vi "Test init device.vi"() -> ()   [LabVIEW 2020]
uses:
  PIC-device/PIC-Device.lvclass
  Toggle 6/Toggle 6.lvclass
  C:/Sandbox/RF Bench/Source Code/WiSpry Test Framework/Devices/PIC-device/PIC-Device.lvclass
panel:
  out "Device out":refnum<class "PIC-Device.lvclass">
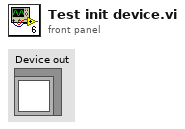
[diagram p1: front panel]
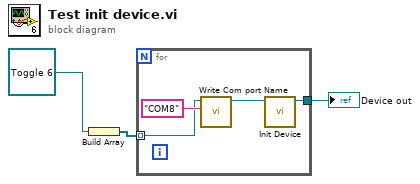
[diagram p0: block diagram]
diagram:
  n1 = Build Array(refnum<class "Toggle 6.lvclass"> refnum ("Toggle 6.lvclass")) -> (w2:refnum<class "Toggle 6.lvclass">[])
  n2 = for {
    tunnel: [w5] -> w1
    tunnel: w2 -> [w4] mode=indexing
    n3 = call-dynamic "Write Com port Name.vi"("Com port Name"="COM8", "Device in"=w4) -> ("Device out"=w6:refnum<class "Toggle 6.lvclass">)  [unwired: 9 in]
    n4 = call-dynamic "Init Device.vi"("Toggle 6 in"=w6) -> ("Toggle 6 out"=w5:refnum<class "Toggle 6.lvclass">)  [unwired: 9 in, 1 out]
  }
  "Device out" <- w1
